vi "channel_set.vi"(8 "error in (no error)":errorcluster, 11 "Thorlabs_OSA300_64 in":refnum<class "OSA300.lvclass">) -> (0 "error out":errorcluster, 3 "Thorlabs_OSA300_64 out":refnum<class "OSA300.lvclass">)   [LabVIEW 2010, in "OSA300.lvclass"]
uses:
  OSA300.lvclass
  OSA.lvclass
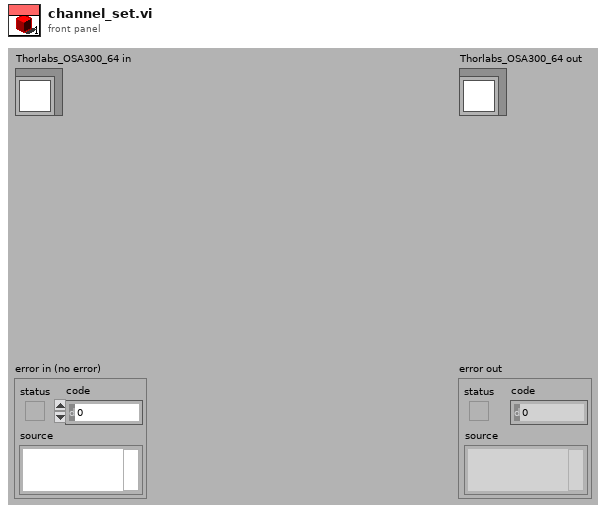
[diagram p1: front panel]
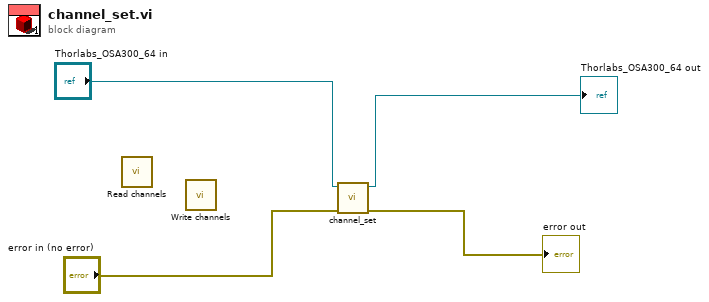
[diagram p0: block diagram]
diagram:
  n1 = call "Read channels.vi"() -> ()  [unwired: 9 in, 3 out]
  n2 = call "Write channels.vi"() -> ()  [unwired: 10 in, 2 out]
  n3 = call-parent "channel_set.vi"("error in (no error)"="error in (no error)", "Thorlabs_OSA_64 in"="Thorlabs_OSA300_64 in") -> ("error out"=→"error out":errorcluster, "Thorlabs_OSA_64 out"=→"Thorlabs_OSA300_64 out":refnum<class "OSA300.lvclass">)  [unwired: 8 in]
